vi "Read Steps.vi"(8 "error in (no error)":errorcluster, 11 "StepCategoryNode in":refnum<class "CleanupCategoryNode.lvclass">) -> (0 "error out":errorcluster, 2 "Steps":refnum<class "Step Config.lvclass">[](array[class]), 3 "StepCategoryNode out":refnum<class "CleanupCategoryNode.lvclass">)   [LabVIEW 2015, in "CleanupCategoryNode.lvclass"]
uses:
  CleanupCategoryNode.lvclass
  Prototype/classes/Step/Config/Step Config.lvclass
  CleanupCategoryNode.lvclass/CleanupCategoryNode.ctl
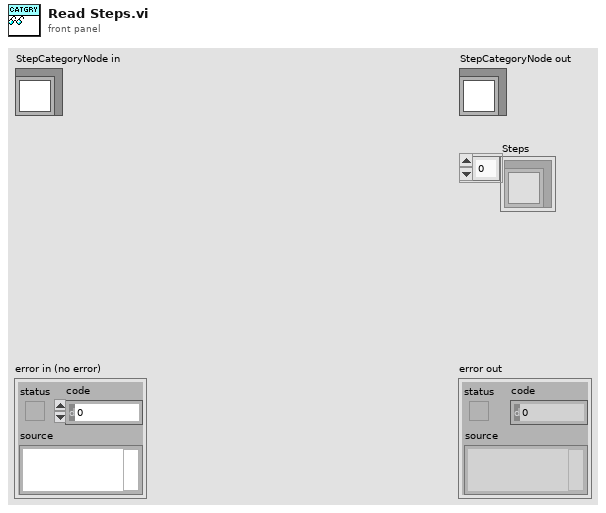
[diagram p1: front panel]
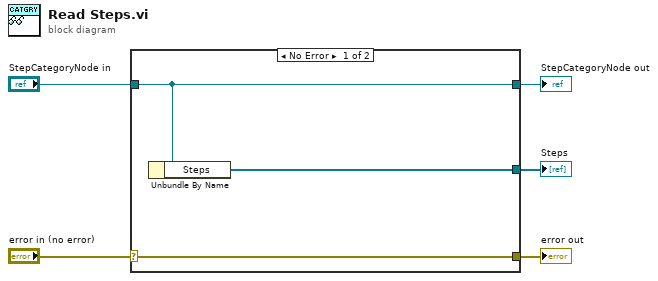
[diagram p0: block diagram]
diagram:
  n1 = case shown="No Error" "error in (no error)" {
    selector: "error in (no error)" -> [w8 w9]
    tunnel: [w8 w9] -> w4
    tunnel: [w7 w10] -> w2
    tunnel: "StepCategoryNode in" -> [w7 w10]
    tunnel: [w6 _] -> w1
    frame No Error {
      n2 = Unbundle By Name(w7) -> ("Steps"=w6:refnum<class "Step Config.lvclass">[])
    }
    frame Error {
    }
  }
  "error out" <- w4
  "StepCategoryNode out" <- w2
  "Steps" <- w1
